vi "Shock&Dyanamics Laboratory - DROPBEAR_June2022_Rev3.vi"() -> ()   [LabVIEW 2019] (continued)
                  }
                }
                n1790 = case shown="True" w2196 {
                  tunnel: [T42."Disabled and Grayed Out" ("Disabled") T42."Enabled" ("Disabled")] -> w2154
                  frame False {
                  }
                  frame True {
                  }
                }
                n1791 = case shown="True" w2197 {
                  tunnel: [T42."Disabled and Grayed Out" ("Disabled") T42."Enabled" ("Disabled")] -> w2153
                  frame False {
                  }
                  frame True {
                  }
                }
                n1792 = case shown="True" w2198 {
                  tunnel: [T42."Disabled and Grayed Out" ("Disabled") T42."Enabled" ("Disabled")] -> w2152
                  frame False {
                  }
                  frame True {
                  }
                }
                n1793 = case shown="True" w2199 {
                  tunnel: [T42."Disabled and Grayed Out" ("Disabled") T42."Enabled" ("Disabled")] -> w2143
                  frame False {
                  }
                  frame True {
                  }
                }
                n1794 = case shown="True" w2200 {
                  tunnel: [T42."Disabled and Grayed Out" ("Disabled") T42."Enabled" ("Disabled")] -> w2142
                  frame False {
                  }
                  frame True {
                  }
                }
                n1795 = case shown="True" w2201 {
                  tunnel: [T42."Disabled and Grayed Out" ("Disabled") T42."Enabled" ("Disabled")] -> w2141
                  frame False {
                  }
                  frame True {
                  }
                }
                n1796 = case shown="True" w2202 {
                  tunnel: [T42."Disabled and Grayed Out" ("Disabled") T42."Enabled" ("Disabled")] -> w2140
                  frame False {
                  }
                  frame True {
                  }
                }
                n1797 = case shown="True" w2138 {
                  tunnel: [T42."Disabled and Grayed Out" ("Disabled") T42."Enabled" ("Disabled")] -> w2119
                  frame False {
                  }
                  frame True {
                  }
                }
                n1798 = case shown="True" w2137 {
                  tunnel: [T42."Disabled and Grayed Out" ("Disabled") T42."Enabled" ("Disabled")] -> w2118
                  frame False {
                  }
                  frame True {
                  }
                }
                n1799 = case shown="True" w2203 {
                  tunnel: [T42."Disabled and Grayed Out" ("Disabled") T42."Enabled" ("Disabled")] -> w2185
                  frame False {
                  }
                  frame True {
                  }
                }
                n1800 = case shown="True" w2188 {
                  tunnel: [T42."Disabled and Grayed Out" ("Disabled") T42."Enabled" ("Disabled")] -> w2176
                  frame False {
                  }
                  frame True {
                  }
                }
                n1801 = property on="PF Chassis 26" class="DigNum (strict)"("DisabledEnum"=w2091) -> (error out=w2089:errorcluster)  [unwired: 2 in, 1 out]
                n1802 = property on="PF Chassis 24" class="DigNum (strict)"("DisabledEnum"=w2097) -> (error out=w2095:errorcluster)  [unwired: 2 in, 1 out]
                n1803 = property on="PF Chassis 28" class="DigNum (strict)"("DisabledEnum"=w2085) -> (error out=w2083:errorcluster)  [unwired: 2 in, 1 out]
                n1804 = property on="PF Chassis 27" class="DigNum (strict)"("DisabledEnum"=w2088) -> (error out=w2086:errorcluster)  [unwired: 2 in, 1 out]
                n1805 = property on="PF Chassis 25" class="DigNum (strict)"("DisabledEnum"=w2094) -> (error out=w2092:errorcluster)  [unwired: 2 in, 1 out]
                n1806 = property on="PF Chassis 29" class="DigNum (strict)"("DisabledEnum"=w2082) -> (error out=w2081:errorcluster)  [unwired: 2 in, 1 out]
                n1807 = property on="PF Chassis 30" class="DigNum (strict)"("DisabledEnum"=w2078) -> (error out=w2080:errorcluster)  [unwired: 2 in, 1 out]
                n1808 = property on="PF Chassis 23" class="DigNum (strict)"("DisabledEnum"=w2100) -> (error out=w2098:errorcluster)  [unwired: 2 in, 1 out]
                n1809 = property on="PF Chassis 31" class="DigNum (strict)"("DisabledEnum"=w2077) -> (error out=w2075:errorcluster)  [unwired: 2 in, 1 out]
                n1810 = property on="PF Chassis 0" class="DigNum (strict)"("DisabledEnum"=w2185) -> (error out=w2187:errorcluster)  [unwired: 2 in, 1 out]
                n1811 = property on="PF Chassis 3" class="DigNum (strict)"("DisabledEnum"=w2178) -> (error out=w2180:errorcluster)  [unwired: 2 in, 1 out]
                n1812 = property on="PF Chassis 20" class="DigNum (strict)"("DisabledEnum"=w2109) -> (error out=w2107:errorcluster)  [unwired: 2 in, 1 out]
                n1813 = property on="PF Chassis 21" class="DigNum (strict)"("DisabledEnum"=w2106) -> (error out=w2104:errorcluster)  [unwired: 2 in, 1 out]
                n1814 = property on="PF Chassis 22" class="DigNum (strict)"("DisabledEnum"=w2103) -> (error out=w2101:errorcluster)  [unwired: 2 in, 1 out]
                n1815 = property on="PF Chassis 1" class="DigNum (strict)"("DisabledEnum"=w2176) -> (error out=w2184:errorcluster)  [unwired: 2 in, 1 out]
                n1816 = property on="PF Chassis 2" class="DigNum (strict)"("DisabledEnum"=w2177) -> (error out=w2182:errorcluster)  [unwired: 2 in, 1 out]
                n1817 = property on="PF Chassis 4" class="DigNum (strict)"("DisabledEnum"=w2173) -> (error out=w2175:errorcluster)  [unwired: 2 in, 1 out]
                n1818 = property on="PF Chassis 18" class="DigNum (strict)"("DisabledEnum"=w2115) -> (error out=w2113:errorcluster)  [unwired: 2 in, 1 out]
                n1819 = property on="PF Chassis 14" class="DigNum (strict)"("DisabledEnum"=w2141) -> (error out=w2147:errorcluster)  [unwired: 2 in, 1 out]
                n1820 = property on="PF Chassis 5" class="DigNum (strict)"("DisabledEnum"=w2164) -> (error out=w2172:errorcluster)  [unwired: 2 in, 1 out]
                n1821 = property on="PF Chassis 6" class="DigNum (strict)"("DisabledEnum"=w2165) -> (error out=w2170:errorcluster)  [unwired: 2 in, 1 out]
                n1822 = property on="PF Chassis 11" class="DigNum (strict)"("DisabledEnum"=w2152) -> (error out=w2157:errorcluster)  [unwired: 2 in, 1 out]
                n1823 = property on="PF Chassis 17" class="DigNum (strict)"("DisabledEnum"=w2118) -> (error out=w2117:errorcluster)  [unwired: 2 in, 1 out]
                n1824 = property on="PF Chassis 7" class="DigNum (strict)"("DisabledEnum"=w2166) -> (error out=w2168:errorcluster)  [unwired: 2 in, 1 out]
                n1825 = property on="PF Chassis 15" class="DigNum (strict)"("DisabledEnum"=w2140) -> (error out=w2145:errorcluster)  [unwired: 2 in, 1 out]
                n1826 = property on="PF Chassis 19" class="DigNum (strict)"("DisabledEnum"=w2112) -> (error out=w2110:errorcluster)  [unwired: 2 in, 1 out]
                n1827 = property on="PF Chassis 8" class="DigNum (strict)"("DisabledEnum"=w2155) -> (error out=w2163:errorcluster)  [unwired: 2 in, 1 out]
                n1828 = property on="PF Chassis 10" class="DigNum (strict)"("DisabledEnum"=w2153) -> (error out=w2159:errorcluster)  [unwired: 2 in, 1 out]
                n1829 = property on="PF Chassis 13" class="DigNum (strict)"("DisabledEnum"=w2142) -> (error out=w2149:errorcluster)  [unwired: 2 in, 1 out]
                n1830 = property on="PF Chassis 9" class="DigNum (strict)"("DisabledEnum"=w2154) -> (error out=w2161:errorcluster)  [unwired: 2 in, 1 out]
                n1831 = property on="PF Chassis 12" class="DigNum (strict)"("DisabledEnum"=w2143) -> (error out=w2151:errorcluster)  [unwired: 2 in, 1 out]
                n1832 = property on="PF Chassis 16" class="DigNum (strict)"("DisabledEnum"=w2119) -> (error out=w2121:errorcluster)  [unwired: 2 in, 1 out]
                n1833 = property on="PF Card 26" class="DigNum (strict)"(error in=w2089, "DisabledEnum"=w2091) -> (error out=w2090:errorcluster)  [unwired: 1 in, 1 out]
                n1834 = property on="PF Card 27" class="DigNum (strict)"(error in=w2086, "DisabledEnum"=w2088) -> (error out=w2087:errorcluster)  [unwired: 1 in, 1 out]
                n1835 = property on="PF Card 25" class="DigNum (strict)"(error in=w2092, "DisabledEnum"=w2094) -> (error out=w2093:errorcluster)  [unwired: 1 in, 1 out]
                n1836 = property on="PF Card 28" class="DigNum (strict)"(error in=w2083, "DisabledEnum"=w2085) -> (error out=w2084:errorcluster)  [unwired: 1 in, 1 out]
                n1837 = property on="PF Card 30" class="DigNum (strict)"(error in=w2080, "DisabledEnum"=w2078) -> (error out=w2079:errorcluster)  [unwired: 1 in, 1 out]
                n1838 = property on="PF Card 24" class="DigNum (strict)"(error in=w2095, "DisabledEnum"=w2097) -> (error out=w2096:errorcluster)  [unwired: 1 in, 1 out]
                n1839 = property on="PF Card 29" class="DigNum (strict)"(error in=w2081, "DisabledEnum"=w2082) -> (error out=w2122:errorcluster)  [unwired: 1 in, 1 out]
                n1840 = property on="PF Card 31" class="DigNum (strict)"(error in=w2075, "DisabledEnum"=w2077) -> (error out=w2076:errorcluster)  [unwired: 1 in, 1 out]
                n1841 = property on="PF Card 22" class="DigNum (strict)"(error in=w2101, "DisabledEnum"=w2103) -> (error out=w2102:errorcluster)  [unwired: 1 in, 1 out]
                n1842 = property on="PF Card 23" class="DigNum (strict)"(error in=w2098, "DisabledEnum"=w2100) -> (error out=w2099:errorcluster)  [unwired: 1 in, 1 out]
                n1843 = property on="PF Card 21" class="DigNum (strict)"(error in=w2104, "DisabledEnum"=w2106) -> (error out=w2105:errorcluster)  [unwired: 1 in, 1 out]
                n1844 = property on="PF Card 20" class="DigNum (strict)"(error in=w2107, "DisabledEnum"=w2109) -> (error out=w2108:errorcluster)  [unwired: 1 in, 1 out]
                n1845 = property on="PF Card 19" class="DigNum (strict)"(error in=w2110, "DisabledEnum"=w2112) -> (error out=w2111:errorcluster)  [unwired: 1 in, 1 out]
                n1846 = property on="PF Card 0" class="DigNum (strict)"(error in=w2187, "DisabledEnum"=w2185) -> (error out=w2186:errorcluster)  [unwired: 1 in, 1 out]
                n1847 = property on="PF Card 18" class="DigNum (strict)"(error in=w2113, "DisabledEnum"=w2115) -> (error out=w2114:errorcluster)  [unwired: 1 in, 1 out]
                n1848 = property on="PF Card 3" class="DigNum (strict)"(error in=w2180, "DisabledEnum"=w2178) -> (error out=w2179:errorcluster)  [unwired: 1 in, 1 out]
                n1849 = property on="PF Card 17" class="DigNum (strict)"(error in=w2117, "DisabledEnum"=w2118) -> (error out=w2116:errorcluster)  [unwired: 1 in, 1 out]
                n1850 = property on="PF Card 1" class="DigNum (strict)"(error in=w2184, "DisabledEnum"=w2176) -> (error out=w2183:errorcluster)  [unwired: 1 in, 1 out]
                n1851 = property on="PF Card 2" class="DigNum (strict)"(error in=w2182, "DisabledEnum"=w2177) -> (error out=w2181:errorcluster)  [unwired: 1 in, 1 out]
                n1852 = property on="PF Card 4" class="DigNum (strict)"(error in=w2175, "DisabledEnum"=w2173) -> (error out=w2174:errorcluster)  [unwired: 1 in, 1 out]
                n1853 = property on="PF Card 14" class="DigNum (strict)"(error in=w2147, "DisabledEnum"=w2141) -> (error out=w2146:errorcluster)  [unwired: 1 in, 1 out]
                n1854 = property on="PF Card 16" class="DigNum (strict)"(error in=w2121, "DisabledEnum"=w2119) -> (error out=w2120:errorcluster)  [unwired: 1 in, 1 out]
                n1855 = property on="PF Card 5" class="DigNum (strict)"(error in=w2172, "DisabledEnum"=w2164) -> (error out=w2171:errorcluster)  [unwired: 1 in, 1 out]
                n1856 = property on="PF Card 6" class="DigNum (strict)"(error in=w2170, "DisabledEnum"=w2165) -> (error out=w2169:errorcluster)  [unwired: 1 in, 1 out]
                n1857 = property on="PF Card 11" class="DigNum (strict)"(error in=w2157, "DisabledEnum"=w2152) -> (error out=w2156:errorcluster)  [unwired: 1 in, 1 out]
                n1858 = property on="PF Card 7" class="DigNum (strict)"(error in=w2168, "DisabledEnum"=w2166) -> (error out=w2167:errorcluster)  [unwired: 1 in, 1 out]
                n1859 = property on="PF Card 15" class="DigNum (strict)"(error in=w2145, "DisabledEnum"=w2140) -> (error out=w2144:errorcluster)  [unwired: 1 in, 1 out]
                n1860 = property on="PF Card 8" class="DigNum (strict)"(error in=w2163, "DisabledEnum"=w2155) -> (error out=w2162:errorcluster)  [unwired: 1 in, 1 out]
                n1861 = property on="PF Card 10" class="DigNum (strict)"(error in=w2159, "DisabledEnum"=w2153) -> (error out=w2158:errorcluster)  [unwired: 1 in, 1 out]
                n1862 = property on="PF Card 13" class="DigNum (strict)"(error in=w2149, "DisabledEnum"=w2142) -> (error out=w2148:errorcluster)  [unwired: 1 in, 1 out]
                n1863 = property on="PF Card 9" class="DigNum (strict)"(error in=w2161, "DisabledEnum"=w2154) -> (error out=w2160:errorcluster)  [unwired: 1 in, 1 out]
                n1864 = property on="PF Card 12" class="DigNum (strict)"(error in=w2151, "DisabledEnum"=w2143) -> (error out=w2150:errorcluster)  [unwired: 1 in, 1 out]
                n1865 = property on="PF Channel 29" class="DigNum (strict)"(error in=w2122, "DisabledEnum"=w2082) -> ()  [unwired: 1 in, 2 out]
                n1866 = property on="PF Channel 0" class="DigNum (strict)"(error in=w2186, "DisabledEnum"=w2185) -> ()  [unwired: 1 in, 2 out]
                n1867 = property on="PF Channel 27" class="DigNum (strict)"(error in=w2087, "DisabledEnum"=w2088) -> ()  [unwired: 1 in, 2 out]
                n1868 = property on="PF Channel 26" class="DigNum (strict)"(error in=w2090, "DisabledEnum"=w2091) -> ()  [unwired: 1 in, 2 out]
                n1869 = property on="PF Channel 28" class="DigNum (strict)"(error in=w2084, "DisabledEnum"=w2085) -> ()  [unwired: 1 in, 2 out]
                n1870 = property on="PF Channel 3" class="DigNum (strict)"(error in=w2179, "DisabledEnum"=w2178) -> ()  [unwired: 1 in, 2 out]
                n1871 = property on="PF Channel 25" class="DigNum (strict)"(error in=w2093, "DisabledEnum"=w2094) -> ()  [unwired: 1 in, 2 out]
                n1872 = property on="PF Channel 21" class="DigNum (strict)"(error in=w2105, "DisabledEnum"=w2106) -> ()  [unwired: 1 in, 2 out]
                n1873 = property on="PF Channel 24" class="DigNum (strict)"(error in=w2096, "DisabledEnum"=w2097) -> ()  [unwired: 1 in, 2 out]
                n1874 = property on="PF Channel 30" class="DigNum (strict)"(error in=w2079, "DisabledEnum"=w2078) -> ()  [unwired: 1 in, 2 out]
                n1875 = property on="PF Channel 1" class="DigNum (strict)"(error in=w2183, "DisabledEnum"=w2176) -> ()  [unwired: 1 in, 2 out]
                n1876 = property on="PF Channel 2" class="DigNum (strict)"(error in=w2181, "DisabledEnum"=w2177) -> ()  [unwired: 1 in, 2 out]
                n1877 = property on="PF Channel 23" class="DigNum (strict)"(error in=w2099, "DisabledEnum"=w2100) -> ()  [unwired: 1 in, 2 out]
                n1878 = property on="PF Channel 22" class="DigNum (strict)"(error in=w2102, "DisabledEnum"=w2103) -> ()  [unwired: 1 in, 2 out]
                n1879 = property on="PF Channel 4" class="DigNum (strict)"(error in=w2174, "DisabledEnum"=w2173) -> ()  [unwired: 1 in, 2 out]
                n1880 = property on="PF Channel 14" class="DigNum (strict)"(error in=w2146, "DisabledEnum"=w2141) -> ()  [unwired: 1 in, 2 out]
                n1881 = property on="PF Channel 20" class="DigNum (strict)"(error in=w2108, "DisabledEnum"=w2109) -> ()  [unwired: 1 in, 2 out]
                n1882 = property on="PF Channel 5" class="DigNum (strict)"(error in=w2171, "DisabledEnum"=w2164) -> ()  [unwired: 1 in, 2 out]
                n1883 = property on="PF Channel 6" class="DigNum (strict)"(error in=w2169, "DisabledEnum"=w2165) -> ()  [unwired: 1 in, 2 out]
                n1884 = property on="PF Channel 11" class="DigNum (strict)"(error in=w2156, "DisabledEnum"=w2152) -> ()  [unwired: 1 in, 2 out]
                n1885 = property on="PF Channel 7" class="DigNum (strict)"(error in=w2167, "DisabledEnum"=w2166) -> ()  [unwired: 1 in, 2 out]
                n1886 = property on="PF Channel 15" class="DigNum (strict)"(error in=w2144, "DisabledEnum"=w2140) -> ()  [unwired: 1 in, 2 out]
                n1887 = property on="PF Channel 17" class="DigNum (strict)"(error in=w2116, "DisabledEnum"=w2118) -> ()  [unwired: 1 in, 2 out]
                n1888 = property on="PF Channel 8" class="DigNum (strict)"(error in=w2162, "DisabledEnum"=w2155) -> ()  [unwired: 1 in, 2 out]
                n1889 = property on="PF Channel 10" class="DigNum (strict)"(error in=w2158, "DisabledEnum"=w2153) -> ()  [unwired: 1 in, 2 out]
                n1890 = property on="PF Channel 13" class="DigNum (strict)"(error in=w2148, "DisabledEnum"=w2142) -> ()  [unwired: 1 in, 2 out]
                n1891 = property on="PF Channel 18" class="DigNum (strict)"(error in=w2114, "DisabledEnum"=w2115) -> ()  [unwired: 1 in, 2 out]
                n1892 = property on="PF Channel 9" class="DigNum (strict)"(error in=w2160, "DisabledEnum"=w2154) -> ()  [unwired: 1 in, 2 out]
                n1893 = property on="PF Channel 19" class="DigNum (strict)"(error in=w2111, "DisabledEnum"=w2112) -> ()  [unwired: 1 in, 2 out]
                n1894 = property on="PF Channel 31" class="DigNum (strict)"(error in=w2076, "DisabledEnum"=w2077) -> ()  [unwired: 1 in, 2 out]
                n1895 = property on="PF Channel 12" class="DigNum (strict)"(error in=w2150, "DisabledEnum"=w2143) -> ()  [unwired: 1 in, 2 out]
                n1896 = property on="PF Channel 16" class="DigNum (strict)"(error in=w2120, "DisabledEnum"=w2119) -> ()  [unwired: 1 in, 2 out]
              }
            }
            n1897 = property on="End Data Recording" class="Bool (strict)"(error in=w33, "Value"=w31) -> (error out=w32:errorcluster)  [unwired: 1 in, 1 out]
          }
          frame "Execute" {
            w2275 = waveform(dbl)[] [] ("array")
            # "Perform Data Aquisition"
            n1898 = property on="Raw Data" class="WFGraph (strict)"(error in=w2276, "Value"=w2275) -> (error out=w2278:errorcluster)  [unwired: 1 in, 1 out]
            n1899 = property on="Longitudinal Strain" class="WFGraph (strict)"(error in=w2278, "Value"=w2275) -> (error out=w2282:errorcluster)  [unwired: 1 in, 1 out]
            n1900 = property on="Bending Strain" class="WFGraph (strict)"(error in=w2282, "Value"=w2275) -> (error out=w2281:errorcluster)  [unwired: 1 in, 1 out]
            n1901 = property on="Longitudinal Strain Rate" class="WFGraph (strict)"(error in=w2281, "Value"=w2275) -> (error out=w2280:errorcluster)  [unwired: 1 in, 1 out]
            n1902 = property on="Velocity" class="WFGraph (strict)"(error in=w2280, "Value"=w2275) -> (error out=w2279:errorcluster)  [unwired: 1 in, 1 out]
            n1903 = property on="Acceleration" class="WFGraph (strict)"(error in=w2279, "Value"=w2275) -> (error out=w2277:errorcluster)  [unwired: 1 in, 1 out]
            n1904 = call "32CHDAQ - Create Channels.vi"("error in"=w2277, "output cluster 2"="output cluster") -> ("error out"=w2284:errorcluster, "task out"=w2285:refnum<k21>)  [unwired: 2 in]
            n1905 = case shown="False" "Trigger (Yes if on)" {
              tunnel: [T6."Continuous" ("View Data") T6."Raw Data" ("View Data")] -> w2269
              frame False {
              }
              frame True {
              }
            }
            n1906 = property on="View Data" class="TabCtl (strict)"("Value"=w2269) -> ()  [unwired: 2 in, 2 out]
            n1907 = case shown="True" "Trigger (Yes if on)" {
              tunnel: w2285 -> [w2323 w2385]
              tunnel: w2284 -> [w2322 w2384]
              tunnel: [w2298 w2364] -> w2273
              tunnel: [w2324 w2363] -> w2272
              tunnel: [w2321 w2358] -> w2271
              tunnel: "output cluster" -> [_ _]
              frame False {
                w2318 = 10123 items=["Finite Samples"=10178, "Continuous Samples"=10123, "Hardware Timed Single Point"=12522]  # Sample Mode
                # "turns all data collected into one waveform"
                # "Wait for task to finish, \nStop the task, and \nClear the task"
                # "Continuous - Record Data"
                n1908 = Multiply(x="Sample Rate (Sa/sec)", y="Timeout (sec) 3") -> (x*y=w2293:dbl)
                n1909 = call-poly <vilib>:"DAQmx Timing.vi"("task/channels in"=w2323, "sample mode"=w2318, "samples per channel"=w2293, "rate"="Sample Rate (Sa/sec)", "source"=tag "OnboardClock" ("Sample Clock Source"), "error in"=w2322) -> ("task out"=w2320:refnum<k21>, "error out"=w2319:errorcluster)  [unwired: 8 in]
                n1910 = property class="DAQmx Timing"(reference=w2320, error in=w2319) -> (reference out=w2307:refnum<k21>, error out=w2315:errorcluster, "SampClk.Rate"=w2290:dbl)
                "Actual Sample Rate (Sa/sec)" <- w2290
                n1911 = property class="DAQmx Task"(reference=w2307) -> ("Channels"=w2306:refnum<k21>[])  [unwired: 1 in, 2 out]
                n1912 = call <vilib>:"DAQmx Start Task.vi"("task/channels in"=w2307, "error in"=w2315) -> ("task out"=w2308:refnum<k21>, "error out"=w2309:errorcluster)  [unwired: 12 in]
                n1913 = Array Size(array=w2306) -> (size(s)=w2288:i32)
                n1914 = Divide(x="Sample Rate (Sa/sec)", y="Refresh Rate") -> (x/y=w2295:dbl)
                n1915 = Round To Nearest(number=w2295) -> (nearest integer value=w2294:dbl)
                n1916 = Divide(x=1.0, y=w2290) -> (x/y=w2291:dbl)
                n1917 = while {
                  tunnel: [w2349] -> w2313
                  shift-right: [w2347] -> w2312
                  shift-left: w2309 -> [w2350]
                  tunnel: "Timeout (sec) 3" -> [w2345]
                  tunnel: w2308 -> [w2343]
                  tunnel: w2294 -> [w2342]
                  tunnel: w2288 -> [_]
                  shift-right: [w2335] -> w2301
                  shift-left: dbl[][] [] -> [w2340]
                  tunnel: w2291 -> [w2332]
                  stop <- w2346 stop-if-true
                  # "adds data and converts to the waveform\none loop at a time"
                  n1918 = call-poly <vilib>:"DAQmx Read.vi"("task/channels in"=w2343, "number of samples per channel"=w2342, "timeout"=w2345, "error in"=w2350) -> ("task out"=w2349:refnum<k21>, "data"=w2339:dbl[][], "error out"=w2347:errorcluster)  [unwired: 9 in]
                  n1919 = Transpose 2D Array(2D array=w2339) -> (transposed array=w2341:dbl[][])
                  n1920 = Build Array (concatenate)(w2340, w2341) -> (w2335:dbl[][])
                  n1921 = Unbundle By Name(w2347) -> ("status"=w2348:bool)
                  n1922 = Or(x=w2348, y="End Data Recording") -> (x .or. y?=w2346:bool)
                  n1923 = Array Size(array=w2335) -> (size(s)=w2337:i32[])
                  n1924 = Index Array(array=w2337, index=1) -> (element=w2336:i32)
                  n1925 = for {
                    N: w2336 -> [_]
                    tunnel: w2335 -> [w2356]
                    shift-right: [w2353] -> w2333
                    shift-left: waveform(dbl)[] [] -> [w2354]
                    tunnel: w2332 -> [w2352]
                    i -> [w2351]
                    n1926 = Index Array(array=w2356, index (col)=w2351) -> (element=w2355:dbl[])  [unwired: 1 in]
                    n1927 = Bundle By Name("dt"=w2352, "Y"=w2355) -> (w2357:waveform(dbl))  [unwired: 1 in]
                    n1928 = Build Array (concatenate)(w2354, w2357) -> (w2353:waveform(dbl)[])
                  }
                  "Waveform Graph" <- w2333
                }
                n1929 = Array Size(array=w2301) -> (size(s)=w2302:i32[])
                n1930 = Index Array(array=w2302, index=1) -> (element=w2303:i32)
                n1931 = for {
                  N: w2303 -> [_]
                  shift-right: [w2331] -> w2298
                  shift-left: waveform(dbl)[] [] ("Raw Data 2") -> [w2329]
                  tunnel: w2301 -> [w2326]
                  tunnel: w2291 -> [w2325]
                  i -> [w2328]
                  n1932 = Index Array(array=w2326, index (col)=w2328) -> (element=w2327:dbl[])  [unwired: 1 in]
                  n1933 = Bundle By Name("dt"=w2325, "Y"=w2327) -> (w2330:waveform(dbl))  [unwired: 1 in]
                  n1934 = Build Array (concatenate)(w2329, w2330) -> (w2331:waveform(dbl)[])
                }
                n1935 = property class="DAQmx Task"(reference=w2313, error in=w2312) -> (reference out=w2296:refnum<k21>, error out=w2297:errorcluster, "Channels"=w2314:refnum<k21>[])
                n1936 = call <vilib>:"DAQmx Stop Task.vi"("task/channels in"=w2296, "error in"=w2297) -> ("task out"=w2311:refnum<k21>, "error out"=w2310:errorcluster)  [unwired: 12 in]
                n1937 = Array Size(array=w2314) -> (size(s)=w2324:i32)
                n1938 = call <vilib>:"DAQmx Clear Task.vi"("task in"=w2311, "error in"=w2310) -> ("error out"=w2321:errorcluster)  [unwired: 13 in]
              }
              frame True {
                w2379 = 10171 items=["Rising"=10280, "Falling"=10171] ("Trigger Slope")
                w2389 = 10050 items=["AC"=10045, "DC"=10050] ("Start.AnlgEdge.Coupling")
                w2390 = 10099 items=["Analog Edge"=10099, "Digital Edge"=10150, "Digital Pattern"=10398, "Analog Window"=10103, "None"=10230] ("Start.TrigType")
                w2395 = 10178 items=["Finite Samples"=10178, "Continuous Samples"=10123, "Hardware Timed Single Point"=12522]  # Sample Mode
                # "Wait for task to finish, \nStop the task, and \nClear the task"
                # "Set Trigger Information"
                # "Set Timing Information"
                # "Timing/Trigger Information"
                # "Timing Settings"
                # "Execute - Record Data"
                n1939 = Bundle("Samples per test (Sa)"="Samples per test (Sa)", "Sample Rate (Sa/sec)"="Sample Rate (Sa/sec)", "Trigger Slope"=w2379, "Trigger Level (V)"="Trigger Level (V)", "Pre-Trigger (%)"=5) -> (w2380:T57)  [unwired: 1 in]
                n1940 = Unbundle(w2380) -> ("Samples per test (Sa)"=w2373:i32, "Sample Rate (Sa/sec)"=w2381:dbl)  [unwired: 3 out]
                n1941 = call-poly <vilib>:"DAQmx Timing.vi"("task/channels in"=w2385, "sample mode"=w2395, "samples per channel"=w2373, "rate"=w2381, "source"=tag "OnboardClock" ("Sample Clock Source"), "error in"=w2384) -> ("task out"=w2397:refnum<k21>, "error out"=w2396:errorcluster)  [unwired: 8 in]
                n1942 = property class="DAQmx Timing"(reference=w2397, error in=w2396) -> (reference out=w2392:refnum<k21>, error out=w2391:errorcluster, "SampClk.Rate"=→"Actual Sample Rate (Sa/sec)":dbl)
                n1943 = Unbundle(w2380) -> ("Samples per test (Sa)"=w2372:i32, "Trigger Slope"=w2378:i32, "Trigger Level (V)"=w2376:dbl, "Pre-Trigger (%)"=w2374:i32)  [unwired: 1 out]
                n1944 = property on="Name (Laser Gate)" class="Str"() -> ("Value"=w2365:string)  [unwired: 2 in, 2 out]
                n1945 = Divide(x=w2374, y=100) -> (x/y=w2387:dbl)
                n1946 = Multiply(x=w2372, y=w2387) -> (x*y=w2386:dbl)
                n1947 = property class="DAQmx Trigger"(reference=w2392, error in=w2391, "Ref.TrigType"=w2390, "Ref.AnlgEdge.Src"=w2365, "Ref.AnlgEdge.Slope"=w2378, "Ref.AnlgEdge.Lvl"=w2376, "Ref.AnlgEdge.Coupling"=w2389, "Ref.PretrigSamples"=w2386) -> (reference out=w2405:refnum<k21>, error out=w2371:errorcluster)
                n1948 = property on="Armed" class="Bool (strict)"(error in=w2371, "Value"=TRUE ("Armed")) -> (error out=w2370:errorcluster)  [unwired: 1 in, 1 out]
                n1949 = call <vilib>:"DAQmx Start Task.vi"("task/channels in"=w2405, "error in"=w2370) -> ("task out"=w2407:refnum<k21>, "error out"=w2406:errorcluster)  [unwired: 12 in]
                n1950 = call-poly <vilib>:"DAQmx Read.vi"("task/channels in"=w2407, "timeout"="Timeout (sec)", "error in"=w2406) -> ("task out"=w2402:refnum<k21>, "data"=w2364:waveform(dbl)[], "error out"=w2368:errorcluster)  [unwired: 10 in]
                n1951 = property on="Armed" class="Bool (strict)"(error in=w2368, "Value"=FALSE ("Armed")) -> (error out=w2367:errorcluster)  [unwired: 1 in, 1 out]
                n1952 = property on="Triggered" class="Bool (strict)"(error in=w2367, "Value"=TRUE ("Triggered")) -> (error out=w2401:errorcluster)  [unwired: 1 in, 1 out]
                n1953 = property class="DAQmx Task"(reference=w2402, error in=w2401) -> (reference out=w2399:refnum<k21>, error out=w2400:errorcluster, "Channels"=w2404:refnum<k21>[])
                n1954 = Array Size(array=w2404) -> (size(s)=w2363:i32)
                n1955 = call <vilib>:"DAQmx Wait Until Done.vi"("task/channels in"=w2399, "timeout (sec)"="Timeout (sec)", "error in"=w2400) -> ("task out"=w2360:refnum<k21>, "error out"=w2359:errorcluster)  [unwired: 11 in]
                n1956 = call <vilib>:"DAQmx Stop Task.vi"("task/channels in"=w2360, "error in"=w2359) -> ("task out"=w2362:refnum<k21>, "error out"=w2361:errorcluster)  [unwired: 12 in]
                n1957 = call <vilib>:"DAQmx Clear Task.vi"("task in"=w2362, "error in"=w2361) -> ("error out"=w2358:errorcluster)  [unwired: 13 in]
              }
            }
            "Raw Data" <- w2273
            "Number of Channels" <- w2272
            n1958 = case shown="Error" w2271 {
              selector: w2271 -> [w2409 w2412]
              tunnel: [32CHDAQ_-_Cases."Process Data" ("Program State") 32CHDAQ_-_Cases."Idle" ("Program State")] -> w2283
              tunnel: [w2409 errorcluster {"status"=FALSE, "code"=0, "source"=""} ("error IO")] -> w2274
              frame No Error {
              }
              frame Error {
                n1959 = flat-sequence {
                  tunnel: w2412 -> [w2414]
                  tunnel: "No Data Was Collected, Please Restart Data Aquisition" ("message") -> [w2418]
                  frame #0 {
                    w2415 = T58 1 items=["no dialog", "OK message", "continue or stop message", "OK message + warnings", "continue/stop + warnings"] ("type of dialog (OK msg:1)")
                    n1960 = call <vilib>:"Simple Error Handler.vi"("type of dialog (OK msg:1)"=w2415, "error in (no error)"=w2414) -> ()  [unwired: 3 in, 5 out]
                  }
                  frame #1 {
                    w2416 = FALSE ("Armed")
                    n1961 = property on="Armed" class="Bool (strict)"("Value"=w2416) -> (error out=w2417:errorcluster)  [unwired: 2 in, 1 out]
                    n1962 = property on="Triggered" class="Bool (strict)"(error in=w2417, "Value"=w2416) -> ()  [unwired: 1 in, 2 out]
                    n1963 = One Button Dialog(message=w2418, button name ("OK")="OK") -> ()  [unwired: 1 out]
                  }
                }
              }
            }
          }
          frame "Process Data" {
            w2452 = "Strain (um/m)" ("Y Scale.Name Label.Text")
            w2477 = TRUE ("Legend:Autosize")
            # "Process and Plot Data"
            # "Velocity Plot"
            # "Acceleration Plot"
            # "Longitudinal Strain Rate"
            # "Bending Strain"
            # "Longitudinal Strain"
            n1964 = property on="Trigger (Yes if on)" class="Bool (strict)"() -> ("Value"=w2423:bool)  [unwired: 2 in, 2 out]
            n1965 = property on="View Data" class="TabCtl (strict)"(error in=w2421, "Value"=T6."Raw Data" ("View Data")) -> (error out=w2420:errorcluster)  [unwired: 1 in, 1 out]
            n1966 = property on="Raw Data" class="WFGraph (strict)"(error in=w2420) -> (error out=w2426:errorcluster, "Value"=w2427:waveform(dbl)[])  [unwired: 1 in, 1 out]
            n1967 = case shown="True" w2423 {
              tunnel: w2427 -> [_ w2512]
              tunnel: [0.0 w2521] -> w2428
              frame False {
              }
              frame True {
                w2514 = -0.2 ("y")
                w2515 = -0.7 ("y")
                w2519 = TRUE ("reset")
                # "Distance covered\nbetween levels"
                # "Level 2"
                # "Level 1"
                n1968 = Index Array(array=w2512, index=0) -> (element=w2503:waveform(dbl))
                n1969 = Multiply(x=w2503, y=-1.0) -> (x*y=w2504:waveform(dbl))
                n1970 = Multiply(x="Extensometer Open Volt (V)", y=w2515) -> (x*y=w2518:dbl)
                n1971 = call-poly <vilib>:"Basic Level Trigger Detection.vi"("signal in"=w2504, "reset"=w2519, "level"=w2518) -> ("trigger location"=w2505:dbl, "error out"=w2520:errorcluster)  [unwired: 10 in, 1 out]
                n1972 = Multiply(x="Extensometer Open Volt (V)", y=w2514) -> (x*y=w2517:dbl)
                n1973 = Multiply(x=0.001, y="Extensometer Gap [mm]") -> (x*y=w2509:dbl)
                n1974 = call-poly <vilib>:"Basic Level Trigger Detection.vi"("signal in"=w2504, "reset"=w2519, "level"=w2517, "error in (no error)"=w2520) -> ("trigger location"=w2506:dbl)  [unwired: 9 in, 2 out]
                n1975 = Subtract(x=w2515, y=w2514) -> (x-y=w2516:dbl)
                n1976 = Multiply(x=w2516, y=w2509) -> (x*y=w2513:dbl)
                n1977 = local read "Sample Rate (Sa/sec)"() -> (w2507:dbl)
                n1978 = Subtract(x=w2506, y=w2505) -> (x-y=w2499:dbl)
                n1979 = Divide(x=w2506, y=w2507) -> (x/y=w2493:dbl)
                n1980 = Divide(x=w2505, y=w2507) -> (x/y=w2497:dbl)
                n1981 = Multiply(x=w2497, y=1000.0 ("x")) -> (x*y=→"t1 [ms]":dbl)
                n1982 = Multiply(x=1000.0, y=w2493) -> (x*y=→"t2 [ms]":dbl)
                n1983 = Multiply(x=-1.0 ("y"), y=w2499) -> (x*y=w2500:dbl)
                n1984 = Divide(x=w2500, y=w2507) -> (x/y=w2522:dbl)
                n1985 = Divide(x=w2513, y=w2522) -> (x/y=w2521:dbl)
              }
            }
            "Striker Velocity (m/s)" <- w2428
            n1986 = property on="output cluster" class="Clust (strict)"(error in=w2426) -> (error out=w2425:errorcluster, "Value"=w2424:T2)  [unwired: 1 in, 1 out]
            n1987 = call "32CHDAQ - Scale Channels.vi"("error in"=w2425, "output cluster 3"=w2424, "Raw Data"=w2427) -> ("error out"=w2478:errorcluster, "Scaled Data"=w2481:waveform(dbl)[])  [unwired: 3 in]
            "Scaled Data" <- w2481
            n1988 = call "32CHDAQ - Seperate Strain 2.vi"("error in"=w2478, "output cluster 4"=w2424, "Scaled Data"=w2481) -> ("error out"=w2479:errorcluster, "Bending Strain Data"=w2461:waveform(dbl)[], "Longitudinal Strain Data"=w2462:waveform(dbl)[])  [unwired: 2 in]
            "Longitudinal Strain" <- w2462
            "Bending Strain" <- w2461
            n1989 = call "32CHDAQ - Strain RateV(1-s).vi"("error in"=w2479, "output cluster 3"=w2424, "Longitudinal Strain Data"=w2462) -> ("error out"=w2480:errorcluster, "Longitudinal Strain Rate Data"=w2483:waveform(dbl)[])  [unwired: 3 in]
            "Longitudinal Strain Rate" <- w2483
            n1990 = call "32CHDAQ - Convert Accel&Vel.vi"("error in"=w2480, "output cluster 3"=w2424, "Scaled Data"=w2481) -> ("error out"=w2490:errorcluster, "Rate Data"=w2484:waveform(dbl)[], "Acceleration data"=w2487:waveform(dbl)[], "Velocity Data"=w2486:waveform(dbl)[])  [unwired: 1 in]
            "Velocity" <- w2486
            "Acceleration" <- w2487
            n1991 = property on="Number of Channels" class="DigNum (strict)"(error in=w2490) -> (error out=w2489:errorcluster, "Value"=w2488:i32)  [unwired: 1 in, 1 out]
            n1992 = Array Size(array=w2487) -> (size(s)=w2442:i32)
            n1993 = Insert Into Array(array=waveform(dbl)[] [], new element #1=w2483, new element #2=w2484) -> (→"Rate Data":waveform(dbl)[])  [unwired: 1 in]
            n1994 = property on="Raw Data" class="WFGraph (strict)"(error in=w2489, "LegNumRows"=w2488) -> (error out=w2472:errorcluster)  [unwired: 1 in, 1 out]
            n1995 = Array Size(array=w2461) -> (size(s)=w2456:i32)
            n1996 = Equal?(x=w2456, y=0) -> (x = y?=w2454:bool)
            n1997 = case shown="False" w2454 {
              tunnel: [T42."Enabled" ("Disabled") T42."Disabled and Grayed Out" ("Disabled")] -> w2453
              frame False {
              }
              frame True {
              }
            }
            n1998 = property on="Longitudinal Strain" class="WFGraph (strict)"(error in=w2472, "LegNumRows"=w2456) -> (error out=w2473:errorcluster)  [unwired: 1 in, 1 out]
            n1999 = property on="Bending Strain" class="WFGraph (strict)"(error in=w2473, "LegNumRows"=w2456) -> (error out=w2474:errorcluster)  [unwired: 1 in, 1 out]
            n2000 = property on="Longitudinal Strain Rate" class="WFGraph (strict)"(error in=w2474, "LegNumRows"=w2456) -> (error out=w2460:errorcluster)  [unwired: 1 in, 1 out]
            n2001 = control-ref of="Longitudinal Strain"() -> (w2467:refnum<vi>)
            n2002 = Array Size(array=w2486) -> (size(s)=w2443:i32)
            n2003 = property on="Property Node" class="WFGraph (strict)"(reference=w2467, error in=w2460, "Disabled"=w2453, "Caption.Text"="", "YScale.NameLbl.Text"=w2452) -> (error out=w2459:errorcluster)  [unwired: 1 out]
            n2004 = control-ref of="Bending Strain"() -> (w2466:refnum<vi>)
            n2005 = control-ref of="Longitudinal Strain Rate"() -> (w2463:refnum<vi>)
            n2006 = property on="Property Node" class="WFGraph (strict)"(reference=w2466, error in=w2459, "Disabled"=w2453, "Caption.Text"="", "YScale.NameLbl.Text"=w2452) -> (error out=w2458:errorcluster)  [unwired: 1 out]
            n2007 = property on="Property Node" class="WFGraph (strict)"(reference=w2463, error in=w2458, "Disabled"=w2453, "Caption.Text"="", "YScale.NameLbl.Text"="Strain Rate (1/s)" ("Y Scale.Name Label.Text")) -> (error out=w2457:errorcluster)  [unwired: 1 out]
            n2008 = Equal?(x=w2443, y=0) -> (x = y?=w2446:bool)
            n2009 = case shown="False" w2446 {
              tunnel: [T42."Enabled" ("Disabled") T42."Disabled and Grayed Out" ("Disabled")] -> w2441
              frame False {
              }
              frame True {
              }
            }
            n2010 = Equal?(x=w2442, y=0) -> (x = y?=w2444:bool)
            n2011 = case shown="False" w2444 {
              tunnel: [T42."Enabled" ("Disabled") T42."Disabled and Grayed Out" ("Disabled")] -> w2440
              frame False {
              }
              frame True {
              }
            }
            n2012 = control-ref of="Velocity"() -> (w2465:refnum<vi>)
            n2013 = property on="Velocity" class="WFGraph (strict)"(error in=w2457, "LegNumRows"=w2443) -> (error out=w2439:errorcluster)  [unwired: 1 in, 1 out]
            n2014 = property on="Property Node" class="WFGraph (strict)"(reference=w2465, error in=w2439, "Disabled"=w2441, "Caption.Text"="", "YScale.NameLbl.Text"="Velocity (m/s)" ("Y Scale.Name Label.Text")) -> (error out=w2438:errorcluster)  [unwired: 1 out]
            n2015 = control-ref of="Acceleration"() -> (w2464:refnum<vi>)
            n2016 = property on="Acceleration" class="WFGraph (strict)"(error in=w2438, "LegNumRows"=w2442) -> (error out=w2437:errorcluster)  [unwired: 1 in, 1 out]
            n2017 = property on="Load Test Data 2" class="Bool"() -> ("Value"=w2431:variant)  [unwired: 2 in, 2 out]
            n2018 = property on="Property Node" class="WFGraph (strict)"(reference=w2464, error in=w2437, "Disabled"=w2440, "Caption.Text"="", "YScale.NameLbl.Text"="Acceleration (g)" ("Y Scale.Name Label.Text")) -> (error out=w2436:errorcluster)  [unwired: 1 out]
            n2019 = property on="Raw Data" class="WFGraph (strict)"(error in=w2436, "LegAutosize"=w2477) -> (error out=w2469:errorcluster)  [unwired: 1 in, 1 out]
            n2020 = property on="Bending Strain" class="WFGraph (strict)"(error in=w2469, "LegAutosize"=w2477) -> (error out=w2470:errorcluster)  [unwired: 1 in, 1 out]
            n2021 = property on="Longitudinal Strain" class="WFGraph (strict)"(error in=w2470, "LegAutosize"=w2477) -> (error out=w2471:errorcluster)  [unwired: 1 in, 1 out]
            n2022 = Variant To Data(type=TRUE, Variant=w2431) -> (data=w2429:bool)  [unwired: 1 in, 1 out]
            n2023 = property on="Longitudinal Strain Rate" class="WFGraph (strict)"(error in=w2471, "LegAutosize"=w2477) -> (error out=w2475:errorcluster)  [unwired: 1 in, 1 out]
            n2024 = case shown="False" w2429 {
              tunnel: [32CHDAQ_-_Cases."Save Data" ("Program State") 32CHDAQ_-_Cases."Idle" ("Program State")] -> w2491
              frame False {
              }
              frame True {
                n2025 = To Variant(anything=FALSE) -> (Variant=w2527:variant)
                n2026 = property on="Load Test Data 2" class="Bool"("Value"=w2527) -> ()  [unwired: 2 in, 2 out]
              }
            }
            n2027 = property on="Velocity" class="WFGraph (strict)"(error in=w2475, "LegAutosize"=w2477) -> (error out=w2476:errorcluster)  [unwired: 1 in, 1 out]
            n2028 = property on="Acceleration" class="WFGraph (strict)"(error in=w2476, "LegAutosize"=w2477) -> (error out=w2468:errorcluster)  [unwired: 1 in, 1 out]
          }
          frame "Save Data" {
            # "Add Dialog Box with Options for 1)other tests, 2)reset test number"
            # "Save Data"
            # "Prompt User to Save Data File"
            n2029 = property on="output cluster" class="Clust (strict)"() -> ("Value"=w2534:T2)  [unwired: 2 in, 2 out]
            n2030 = Two Button Dialog(message="Save Data File?", 1:"No" ("F button name (\"Cancel\")"), 2:"Yes" ("T button name (\"OK\")")) -> (T button?=w2535:bool)
            n2031 = case shown="True" w2535 {
              tunnel: [w2547 w2574] -> w2543
              tunnel: errorcluster {"status"=FALSE, "code"=0, "source"=""} ("error out") -> [w2547 w2558]
              tunnel: w2534 -> [_ w2573]
              frame False {
              }
              frame True {
                # "Save Scaled Data / First Pulse of Scaled Data"
